vi "Do.vi"(8 "error in (no error)":errorcluster, 10 "Actor in":refnum<class "Actor.lvclass">, 11 "Sub Panel Insertion Msg":refnum<class "Sub Panel Insertion Msg.lvclass">) -> (0 "error out":errorcluster, 2 "Actor out":refnum<class "Actor.lvclass">)   [LabVIEW 2020, in "Msg.lvlib" / "Sub Panel Insertion Msg.lvclass"]
doc: "This Do implementation will insert the front panel of the active actor core clone VI in a sub panel if the sub panel reference is valid.\n\nThe Sub panel reference is closed if requested."
uses:
  Sub Panel Insertion Msg.lvclass
  PPL/HDH.Actor Framework.Core.Actor.lvlibp/1abvi3w/vi.lib/ActorFramework/Actor/Actor.lvclass
  Sub Panel Insertion Msg.lvclass/Sub Panel Insertion Msg.ctl
  Msg.lvlib
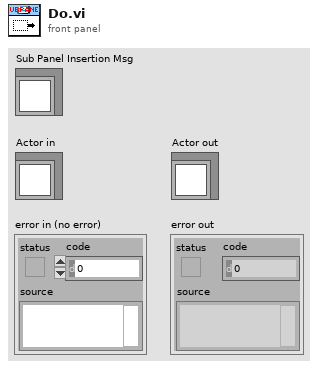
[diagram p1: front panel]
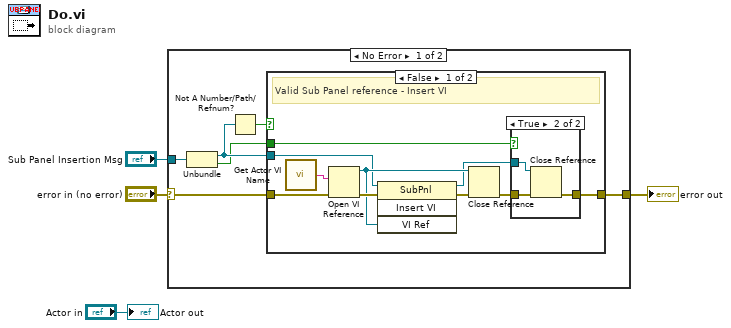
[diagram p0: block diagram]
diagram:
  n1 = case shown="No Error" "error in (no error)" {
    selector: "error in (no error)" -> [w10 w26]
    tunnel: [w9 w26] -> w4
    tunnel: "Sub Panel Insertion Msg" -> [w8 _]
    frame No Error {
      n2 = Unbundle(w8) -> (w7:refnum<vi>, w5:bool)
      n3 = Not A Number/Path/Refnum?(number/path/refnum=w7) -> (NaN/Path/Refnum?=w6:bool)
      n4 = case shown="False" w6 {
        tunnel: w10 -> [w19 w25]
        tunnel: [w12 w25] -> w9
        tunnel: w7 -> [w15 _]
        tunnel: w5 -> [w14 _]
        frame False {
          # "Valid Sub Panel reference - Insert VI"
          n5 = call "Get Actor VI Name.vi"() -> ("Actor VI Name"=w20:string)
          n6 = Open VI Reference(vi path=w20, error in (no error)=w19) -> (vi reference=w16:refnum<vi>, error out=w18:errorcluster)  [unwired: 4 in]
          n7 = invoke class="SubPnl" method="Insert VI"(reference=w15, error in=w18, "VI Ref"=w16) -> (reference out=w11:refnum<vi>, error out=w17:errorcluster)  [unwired: 1 in, 2 out]
          n8 = Close Reference(reference=w16, error in (no error)=w17) -> (error out=w13:errorcluster)
          n9 = case shown="True" w14 {
            tunnel: w13 -> [w21 w24]
            tunnel: [w21 w23] -> w12
            tunnel: w11 -> [_ w22]
            frame False {
            }
            frame True {
              n10 = Close Reference(reference=w22, error in (no error)=w24) -> (error out=w23:errorcluster)
            }
          }
        }
        frame True {
          # "Invalid Sub Panel reference - Abort operation"
        }
      }
    }
    frame Error {
    }
  }
  "error out" <- w4
  "Actor out" <- "Actor in"
